vi "Hardware-DI-Scope-Host.vi"() -> ()   [LabVIEW 2016]
uses:
  <vilib>/Powertrain Controls/Device Drivers/DCM/DI/FPGA/Capture Event.ctl
  <vilib>/Powertrain Controls/Device Drivers/DCM/Rev0/FPGA/DI - ADC Signals.ctl
  <vilib>/Utility/miscctls.llb/LVPositionTypeDef.ctl
  <vilib>/Powertrain Controls/Device Drivers/DCM/DI/FPGA/DCM - FPGA - DI.lvlib
  <vilib>/Powertrain Controls/Device Drivers/DCM/Rev0/FPGA/DCM - FPGA.lvlib
panel:
  in  "Length":sgl=0.01 caption="[s]" min=0 max=0.055 format="%#_6p"
  in  "ScopeEnable":bool
  in  "ScopeEvent":u8(ring) items=["Unused", "Injector A1", "Injector A2", "Injector A3", "Injector A4", "Injector A5", "Injector A6", "Injector A7", "Injector A8/PumpA", "Injector B1", "Injector B2", "Injector B3", "Injector B4", "Injector B5", "Injector B6", "Injector B7", "Injector B8/PumpB", "User OS", "Diff IO 1", "Diff IO 2", "Diff IO 3", "Diff IO 4", "Diff IO 5", "Diff IO 6", "Diff IO 7", "Diff IO 8", "Aux 1", "Aux 2", "Aux 3", "Aux 4", "Aux 5", "Aux 6", "Aux 7", "Aux 8", "Aux 9", "Aux 10", "Aux 11", "Aux 12", "Aux 13", "Aux 14", "Aux 15", "Aux 16"]
  out "dt":sgl
  in  "_DI ADC Select":T1
  in  "_DI Scope Event":T2
  in  "ChanSelect4":u8(ring) items=["I LS A1/A5", "I LS A2/A6", "I LS A3/A7", "I LS A4", "I LS A8/PumpA", "V PZ A1", "V PZ A2", "V PZ A3", "V PZ A4", "V S A1", "V S A2", "V S A3", "V S A4", "V S A5", "V S A6", "V S A7", "V S A8", "V Pump A", "V Secondary A1A2", "V Secondary A3A4", "V Ext HV A", "------------------------ ", "I LS B1/B5", "I LS B2/B6", "I LS B3/B7", "I LS B4", "I LS B8/PumpB", "V PZ B1", "V PZ B2", "V PZ B3", "V PZ B4", "V S B1", "V S B2", "V S B3", "V S B4", "V S B5", "V S B6", "V S B7", "V S B8", "V Pump B", "V Secondary B1B2", "V Secondary B3B4", "V Ext HV B", "-------------------------  ", "AI 1", "AI 2", "AI 3", "AI 4", "AI 5", "AI 6", "AI 7", "AI 8", "AI 9", "AI 10", "AI 11", "AI 12", "-------------------------   ", "V DRVP"]
  in  "ChanSelect3":u8(ring) items=["I LS A1/A5", "I LS A2/A6", "I LS A3/A7", "I LS A4", "I LS A8/PumpA", "V PZ A1", "V PZ A2", "V PZ A3", "V PZ A4", "V S A1", "V S A2", "V S A3", "V S A4", "V S A5", "V S A6", "V S A7", "V S A8", "V Pump A", "V Secondary A1A2", "V Secondary A3A4", "V Ext HV A", "------------------------ ", "I LS B1/B5", "I LS B2/B6", "I LS B3/B7", "I LS B4", "I LS B8/PumpB", "V PZ B1", "V PZ B2", "V PZ B3", "V PZ B4", "V S B1", "V S B2", "V S B3", "V S B4", "V S B5", "V S B6", "V S B7", "V S B8", "V Pump B", "V Secondary B1B2", "V Secondary B3B4", "V Ext HV B", "-------------------------  ", "AI 1", "AI 2", "AI 3", "AI 4", "AI 5", "AI 6", "AI 7", "AI 8", "AI 9", "AI 10", "AI 11", "AI 12", "-------------------------   ", "V DRVP"]
  in  "ChanSelect2":u8(ring) items=["I LS A1/A5", "I LS A2/A6", "I LS A3/A7", "I LS A4", "I LS A8/PumpA", "V PZ A1", "V PZ A2", "V PZ A3", "V PZ A4", "V S A1", "V S A2", "V S A3", "V S A4", "V S A5", "V S A6", "V S A7", "V S A8", "V Pump A", "V Secondary A1A2", "V Secondary A3A4", "V Ext HV A", "------------------------ ", "I LS B1/B5", "I LS B2/B6", "I LS B3/B7", "I LS B4", "I LS B8/PumpB", "V PZ B1", "V PZ B2", "V PZ B3", "V PZ B4", "V S B1", "V S B2", "V S B3", "V S B4", "V S B5", "V S B6", "V S B7", "V S B8", "V Pump B", "V Secondary B1B2", "V Secondary B3B4", "V Ext HV B", "-------------------------  ", "AI 1", "AI 2", "AI 3", "AI 4", "AI 5", "AI 6", "AI 7", "AI 8", "AI 9", "AI 10", "AI 11", "AI 12", "-------------------------   ", "V DRVP"]
  in  "ChanSelect1":u8(ring) items=["I LS A1/A5", "I LS A2/A6", "I LS A3/A7", "I LS A4", "I LS A8/PumpA", "V PZ A1", "V PZ A2", "V PZ A3", "V PZ A4", "V S A1", "V S A2", "V S A3", "V S A4", "V S A5", "V S A6", "V S A7", "V S A8", "V Pump A", "V Secondary A1A2", "V Secondary A3A4", "V Ext HV A", "------------------------ ", "I LS B1/B5", "I LS B2/B6", "I LS B3/B7", "I LS B4", "I LS B8/PumpB", "V PZ B1", "V PZ B2", "V PZ B3", "V PZ B4", "V S B1", "V S B2", "V S B3", "V S B4", "V S B5", "V S B6", "V S B7", "V S B8", "V Pump B", "V Secondary B1B2", "V Secondary B3B4", "V Ext HV B", "-------------------------  ", "AI 1", "AI 2", "AI 3", "AI 4", "AI 5", "AI 6", "AI 7", "AI 8", "AI 9", "AI 10", "AI 11", "AI 12", "-------------------------   ", "V DRVP"]
  out "Data":sgl[][](graph)
  in  "Snapshot":bool
  in  "SnapshotFile":string caption="User VI File Path (.vi relative to default data directory)"
  # "Snapshot File Path (.tdms relative to default data directory)"
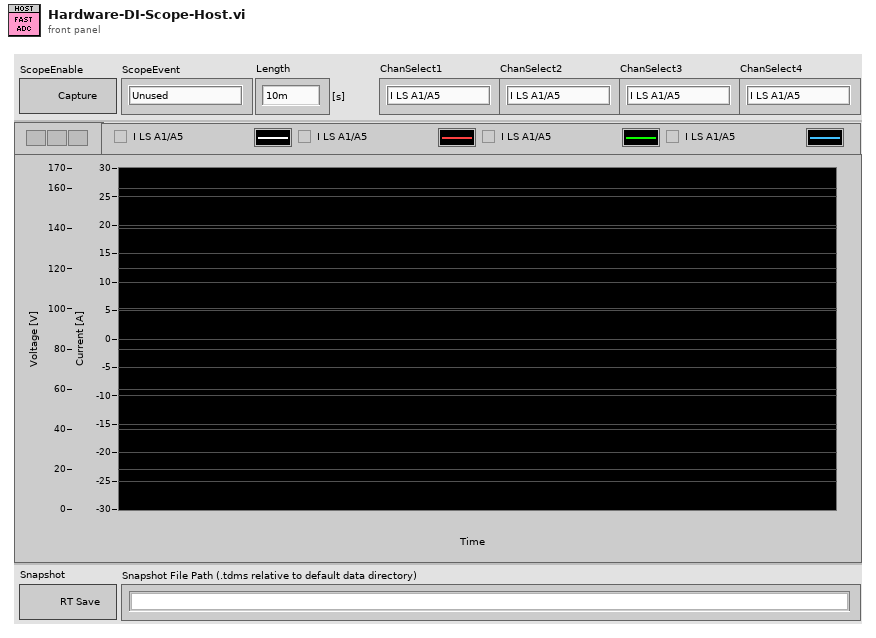
[diagram p1: front panel]
types:
  T1 = typedef "DCM - FPGA.lvlib/DI - ADC Signals.ctl" = enum8{"I LS A1/A5", "I LS A2/A6", "I LS A3/A7", "I LS A4", "I LS A8/PumpA", "V PZ A1", "V PZ A2", "V PZ A3", "V PZ A4", "V S A1", "V S A2", "V S A3", "V S A4", "V S A5", "V S A6", "V S A7", "V S A8", "V Pump A", "V Secondary A1A2", "V Secondary A3A4", "V Ext HV A", "------------------------ ", "I LS B1/B5", "I LS B2/B6", "I LS B3/B7", "I LS B4", "I LS B8/PumpB", "V PZ B1", "V PZ B2", "V PZ B3", "V PZ B4", "V S B1", "V S B2", "V S B3", "V S B4", "V S B5", "V S B6", "V S B7", "V S B8", "V Pump B", "V Secondary B1B2", "V Secondary B3B4", "V Ext HV B", "-------------------------  ", "AI 1", "AI 2", "AI 3", "AI 4", "AI 5", "AI 6", "AI 7", "AI 8", "AI 9", "AI 10", "AI 11", "AI 12", "-------------------------   ", "V DRVP"}
  T2 = typedef "DCM - FPGA - DI.lvlib/Capture Event.ctl" = enum8{"Unused", "Injector A1", "Injector A2", "Injector A3", "Injector A4", "Injector A5", "Injector A6", "Injector A7", "Injector A8/PumpA", "Injector B1", "Injector B2", "Injector B3", "Injector B4", "Injector B5", "Injector B6", "Injector B7", "Injector B8/PumpB", "User OS", "Diff IO 1", "Diff IO 2", "Diff IO 3", "Diff IO 4", "Diff IO 5", "Diff IO 6", "Diff IO 7", "Diff IO 8", "Aux 1", "Aux 2", "Aux 3", "Aux 4", "Aux 5", "Aux 6", "Aux 7", "Aux 8", "Aux 9", "Aux 10", "Aux 11", "Aux 12", "Aux 13", "Aux 14", "Aux 15", "Aux 16"}
  T3 = typedef "LVPositionTypeDef.ctl" = cluster{"Left":i32, "Top":i32}
  T4 = typedef "LVStringsAndValuesArrayTypeDef_U8.ctl" = cluster{"String":string, "Value":u8}[]
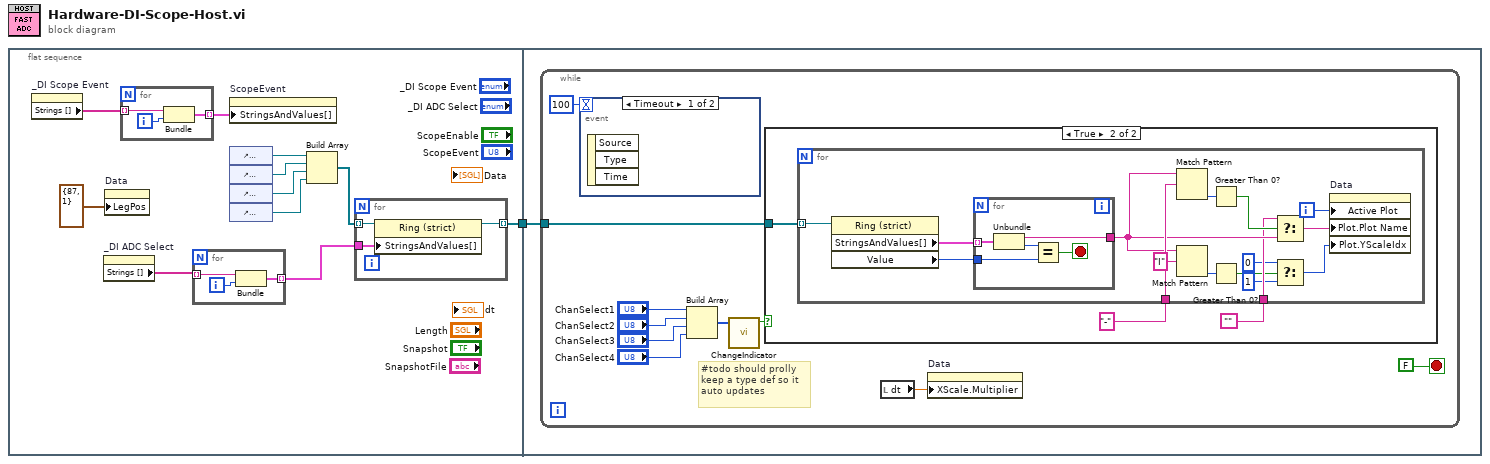
[diagram p0: block diagram]
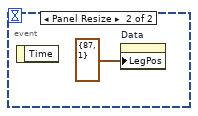
[diagram p2: hidden frame]
diagram:
  n1 = flat-sequence {
    tunnel: [w3] -> w1
    tunnel: w1 -> [w22]
    frame #0 {
      n2 = property on="_DI Scope Event" class="Enum (strict)"() -> ("Strings []"=w11:string[])  [unwired: 2 in, 2 out]
      n3 = property on="_DI ADC Select" class="Enum (strict)"() -> ("Strings []"=w6:string[])  [unwired: 2 in, 2 out]
      n4 = property on="Data" class="WFGraph (strict)"("LegPos"=T3 {"Left"=87, "Top"=1} ("Legend:Position")) -> ()  [unwired: 2 in, 2 out]
      n5 = for {
        tunnel: w11 -> [w21] mode=indexing
        tunnel: [w19] -> w12 mode=indexing
        i -> [w20]
        n6 = Bundle(w21, w20) -> (w19:cluster{string, i32})  [unwired: 1 in]
      }
      n7 = for {
        tunnel: w6 -> [w18] mode=indexing
        tunnel: [w16] -> w4 mode=indexing
        i -> [w17]
        n8 = Bundle(w18, w17) -> (w16:cluster{string, i32})  [unwired: 1 in]
      }
      n9 = property on="ScopeEvent" class="Ring (strict)"("StringsAndValues[]"=w12) -> ()  [unwired: 2 in, 2 out]
      n10 = control-ref of="ChanSelect1"() -> (w7:refnum<vi>)
      n11 = control-ref of="ChanSelect2"() -> (w8:refnum<vi>)
      n12 = control-ref of="ChanSelect3"() -> (w9:refnum<vi>)
      n13 = control-ref of="ChanSelect4"() -> (w10:refnum<vi>)
      n14 = Build Array(w7, w8, w9, w10) -> (w5:refnum<vi>[])
      n15 = for {
        tunnel: w5 -> [w15] mode=indexing
        tunnel: w4 -> [w14]
        tunnel: [w13] -> w3 mode=indexing
        n16 = property on="Property Node" class="Ring (strict)"(reference=w15, "StringsAndValues[]"=w14) -> (reference out=w13:refnum<vi>)  [unwired: 1 in, 1 out]
      }
    }
    frame #1 {
      n17 = while {
        tunnel: w22 -> [w25]
        stop <- FALSE stop-if-true
        # "#todo should prolly\nkeep a type def so it \nauto updates"
        n18 = event shown="[0] Timeout" {
          selector: _ -> [_ _]
          dyn-events: _ -> [_ _]
          timeout: 100 -> [_ _]
          event Timeout {
            n19 = event-data() -> ()  [unwired: 1 in, 3 out]
          }
          event Panel Resize {
            n20 = event-data() -> ()  [unwired: 1 in, 1 out]
            n21 = property on="Data" class="WFGraph (strict)"("LegPos"=T3 {"Left"=87, "Top"=1} ("Legend:Position")) -> ()  [unwired: 2 in, 2 out]
          }
        }
        n22 = Build Array("ChanSelect1", "ChanSelect2", "ChanSelect3", "ChanSelect4") -> (w26:u8[])
        n23 = call "ChangeIndicator.vi"("Input"=w26) -> ("Change"=w31:bool)  [unwired: 9 in]
        n24 = case shown="True" w31 {
          tunnel: w25 -> [_ w36]
          frame False {
          }
          frame True {
            n25 = for {
              tunnel: "" -> [w41]
              tunnel: "-" ("regular expression") -> [w49]
              tunnel: w36 -> [w46] mode=indexing
              i -> [w45]
              n26 = property on="Property Node" class="Ring (strict)"(reference=w46) -> ("StringsAndValues[]"=w48:T4, "Value"=w47:u8)  [unwired: 1 in, 2 out]
              n27 = for {
                tunnel: w48 -> [w57] mode=indexing
                tunnel: [w54] -> w44
                tunnel: w47 -> [w53]
                stop <- w55 stop-if-true
                n28 = Unbundle(w57) -> ("String"=w54:string, "Value"=w56:u8)
                n29 = Equal?(x=w56, y=w53) -> (x = y?=w55:bool)
              }
              n30 = Match Pattern(string=w44, regular expression=w49) -> (offset past match=w52:i32)  [unwired: 1 in, 3 out]
              n31 = Match Pattern(string=w44, regular expression="I") -> (offset past match=w42:i32)  [unwired: 1 in, 3 out]
              n32 = Greater Than 0?(x=w52) -> (x > 0?=w51:bool)
              n33 = Greater Than 0?(x=w42) -> (x > 0?=w40:bool)
              n34 = Select(t=w41, s=w51, f=w44) -> (s? t:f=w50:string)
              n35 = Select(t=u32 0, s=w40, f=u32 1 ("t")) -> (s? t:f=w37:u32)
              n36 = property on="Data" class="WFGraph (strict)"("Active Plot"=w45, "Plot.Plot Name"=w50, "Plot.YScaleIdx"=w37) -> ()  [unwired: 2 in, 2 out]
            }
          }
        }
        n37 = local read "dt"() -> (w23:sgl)
        n38 = property on="Data" class="WFGraph (strict)"("XScale.Multiplier"=w23) -> ()  [unwired: 2 in, 2 out]
      }
    }
  }
